vi "Acourse_Water-Props_clean.vi"(8 "error in":errorcluster, 11 "Water Avg (°F)":dbl) -> (0 "error out":errorcluster, 1 "Density (lbm/ft³)":dbl, 2 "mu (lbm/ft*s)":dbl, 3 "Cp (BTU/lbm°F)":dbl)   [LabVIEW 2016]
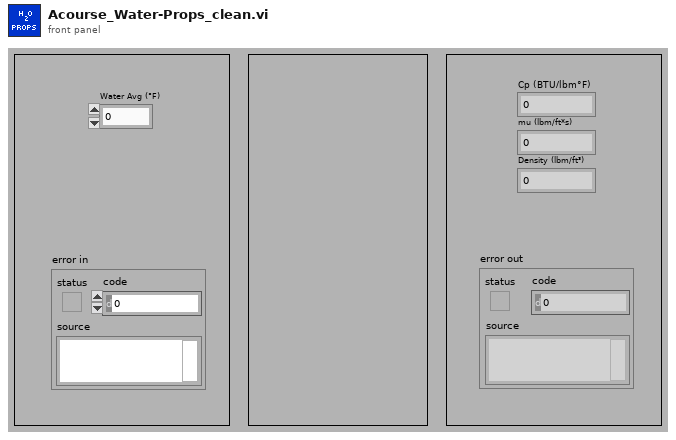
[diagram p1: front panel]
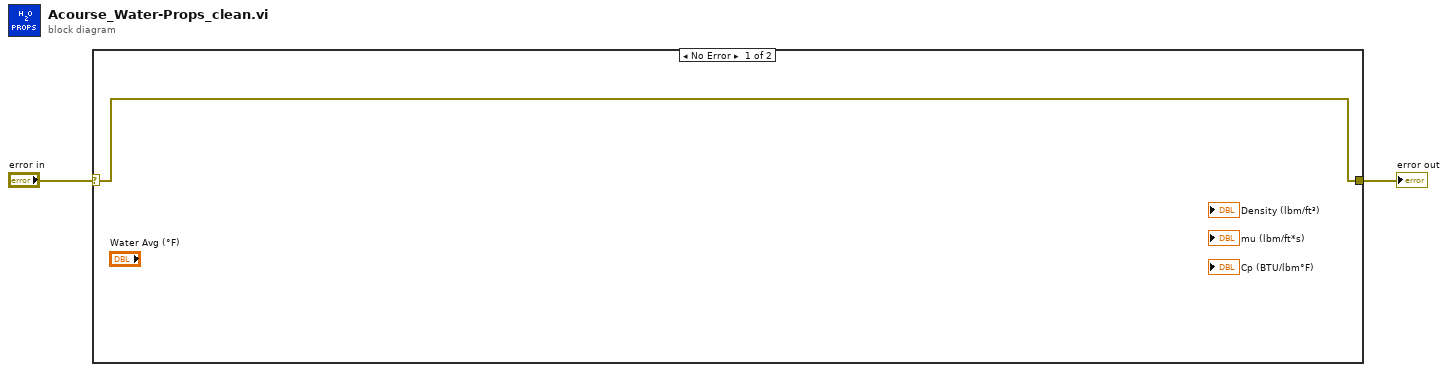
[diagram p0: block diagram]
diagram:
  n1 = case shown="No Error" "error in" {
    selector: "error in" -> [w3 w4]
    tunnel: [w3 w4] -> w1
    frame No Error {
    }
    frame Error {
    }
  }
  "error out" <- w1
